vi "SimpleWatson.vi"(9 "APIKey":string, 11 "Image":path=path "/Users/crogers/Desktop/AllThingsLEGO/AI/Ziyi/imageTest") -> (0 "score":dbl, 1 "guess":string, 3 "image sent":picture)   [LabVIEW 2019]
panel:
  # "Directions\n1. sign up for a watson account : https://www.ibm.com/watson \n     a. confirm through email\n2. open up https://cloud.ibm.com\n    a. go to menu\n    b. Find Watson\n    c. Go to Browse Services\n    d. Choose Visual Recognition \n    e. Create a Lite plan - go to Manage - and read the API key\n    f. OR if you already have a plan, go your Watson, \n       Browse Existing Services and select you visiton recognition\n       service and get your API Key\n3. Test it out\n    a. go to https://cloud.ibm.com\n    b. go to menu, Watson\n    c. select Existing Services\n    d. select watson-vision-combined service\n    e. Launch Watson Studio\n    f. select the Food model\n    g. grab an image from the web and see if it can be identified"
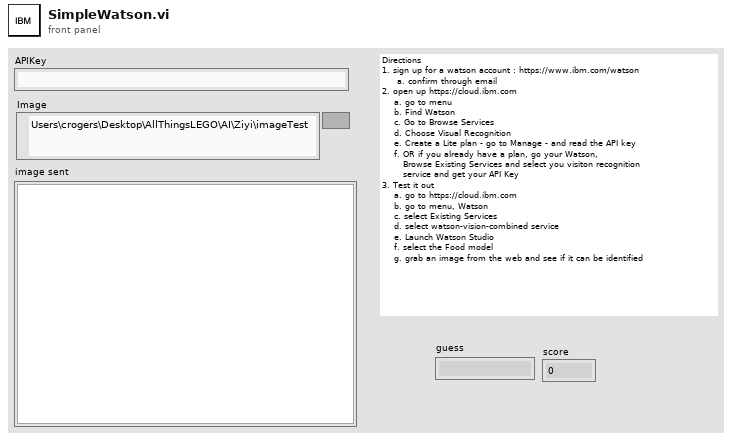
[diagram p1: front panel]
types:
  T1 = typedef "imagedata.ctl" = cluster{"image type":i32, "image depth":i32, "image":u8[], "mask":u8[], "colors":u32[], "Rectangle":cluster{"left":i16, "top":i16, "right":i16, "bottom":i16}}
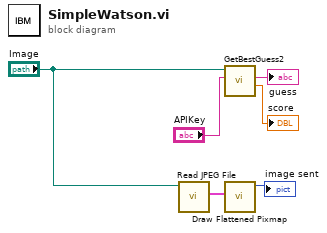
[diagram p0: block diagram]
diagram:
  n1 = call <vilib>:"Read JPEG File.vi"("path to JPEG file"="Image") -> ("image data"=w2:T1)  [unwired: 8 in, 2 out]
  n2 = call "GetBestGuess2.vi"("APIKey"="APIKey", "Image"="Image") -> ("score"=→"score":dbl, "class"=→"guess":string)  [unwired: 7 in, 1 out]
  n3 = call <vilib>:"Draw Flattened Pixmap.vi"("image data"=w2) -> ("new picture"=→"image sent":picture)  [unwired: 8 in]
